vi "Facade.vi"(0 "Data In":T4, 2 "Display State In":T2, 3 "Container State":T3) -> (6 "Data Out":T4, 7 "Display State Out":T2, 8 "Action":T1)   [LabVIEW 2019, in "XTextCode.xctl"]
uses:
  XTextCode.xctl
  Data.ctl
  <vilib>/_xctls/Container State.ctl
  State.ctl
  <vilib>/_xctls/Action.ctl
  <vilib>/_xctls/XControlSupport.lvlib
  System.Windows.Forms
panel:
  in  "RichTextBox":refnum<k24>(container)
types:
  T1 = typedef "XControlSupport.lvlib/Action.ctl" = cluster{"Data Changed?":bool, "State Changed?":bool, "Action Name":string}
  T2 = typedef "XTextCode.xctl/State.ctl" = cluster{"String":string}
  T3 = typedef "XControlSupport.lvlib/Container State.ctl" = cluster{"Indicator?":bool, "Run Mode?":bool, " Refnum":refnum<vi>}
  T4 = typedef "XTextCode.xctl/Data.ctl" = string
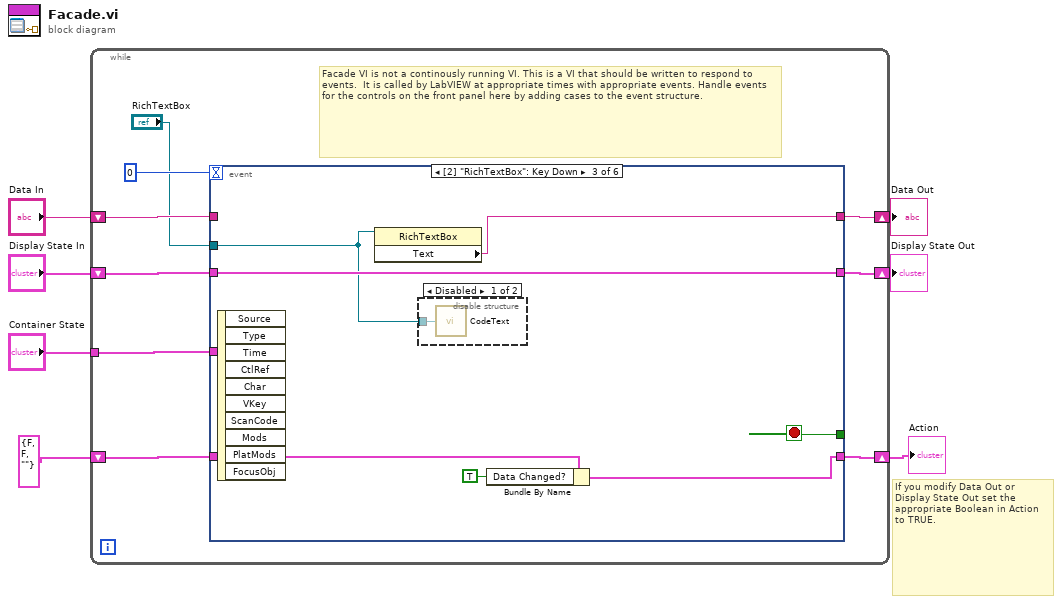
[diagram p0: block diagram]
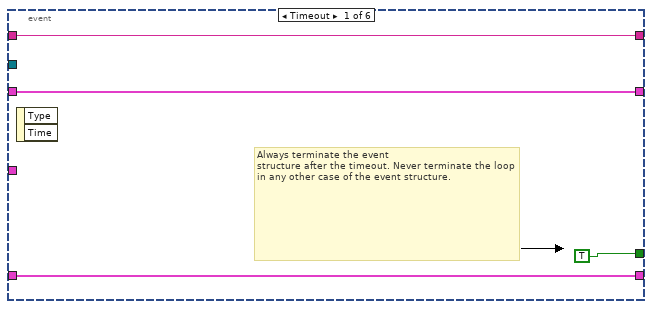
[diagram p2: hidden frame]
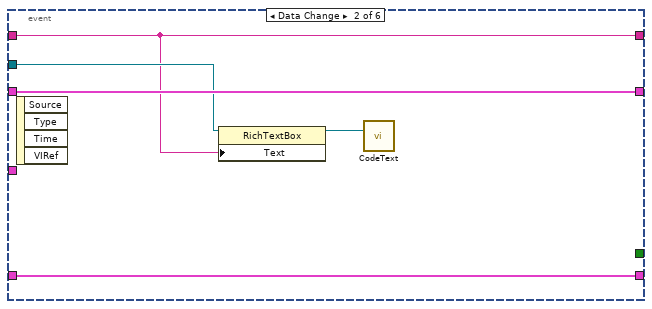
[diagram p3: hidden frame]
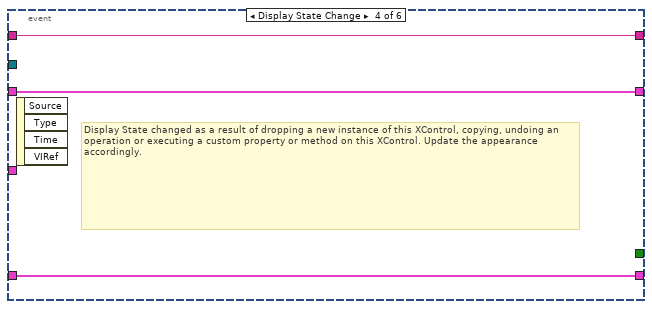
[diagram p5: hidden frame]
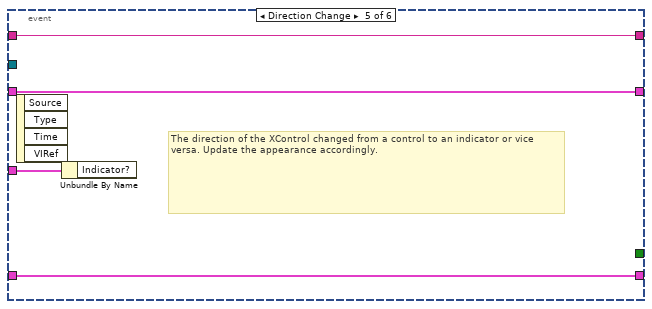
[diagram p6: hidden frame]
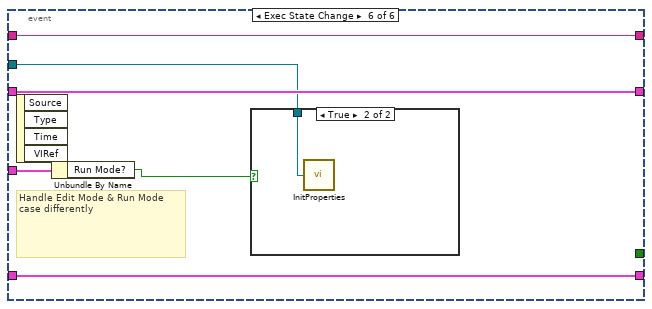
[diagram p7: hidden frame]
diagram:
  # "If you modify Data Out or\nDisplay State Out set the\nappropriate Boolean in Action\nto TRUE."
  n1 = while {
    shift-right: [w16] -> w4
    shift-left: "Display State In" -> [w17]
    tunnel: "Container State" -> [w13]
    shift-right: [w11] -> w7
    shift-left: "Data In" -> [w12]
    shift-right: [w9] -> w2
    shift-left: T1 {"Data Changed?"=FALSE, "State Changed?"=FALSE, "Action Name"=""} ("Action") -> [w10]
    stop <- w15 stop-if-true
    # "Facade VI is not a continously running VI. This is a VI that should be written to respond to events.  It is called by LabVIEW at appropriate times with appropriate events. Handle events for the controls on the front panel here by adding cases to the event structure."
    n2 = event shown="[2] \"RichTextBox\": Key Down" {
      selector: _ -> [_ _ _ _ _ _]
      dyn-events: _ -> [_ _ _ _ _ _]
      timeout: 0 -> [_ _ _ _ _ _]
      tunnel: w17 -> [w19 w26 w32 w36 w39 w45]
      tunnel: [w19 w26 w32 w36 w39 w45] -> w16
      tunnel: [TRUE _ _ _ _ _] -> w15
      tunnel: w13 -> [_ _ _ _ w40 w46]
      tunnel: w12 -> [w18 w23 _ w35 w38 w44]
      tunnel: [w18 w23 w30 w35 w38 w44] -> w11
      tunnel: [w20 w25 w28 w34 w37 w43] -> w9
      tunnel: w10 -> [w20 w25 w29 w34 w37 w43]
      tunnel: "RichTextBox" -> [_ w24 w31 _ _ w41]
      event Timeout {
        # "Always terminate the event\nstructure after the timeout. Never terminate the loop in any other case of the event structure."
        n3 = event-data() -> ()  [unwired: 1 in, 2 out]
      }
      event Data Change {
        n4 = event-data() -> ()  [unwired: 1 in, 4 out]
        n5 = property class="RichTextBox"(reference=w24, "Text"=w23) -> (reference out=w22:refnum<k24>)  [unwired: 1 in, 1 out]
        n6 = call "CodeText.vi"("Seq script"=w22) -> ()
      }
      event "RichTextBox": Key Down {
        n7 = event-data() -> ()  [unwired: 1 in, 10 out]
        n8 = property class="RichTextBox"(reference=w31) -> ("Text"=w30:string)  [unwired: 1 in, 2 out]
        n9 = disable-structure shown="Disabled" {
          disable-tunnel: w31 -> [w33 _]
          frame Disabled {
            n10 = call "CodeText.vi"("Seq script"=w33) -> ()
          }
          frame Enabled {
          }
        }
        n11 = Bundle By Name(cluster=w29, "Data Changed?"=TRUE) -> (w28:T1)
      }
      event Display State Change {
        # "Display State changed as a result of dropping a new instance of this XControl, copying, undoing an operation or executing a custom property or method on this XControl. Update the appearance accordingly."
        n12 = event-data() -> ()  [unwired: 1 in, 4 out]
      }
      event Direction Change {
        # "The direction of the XControl changed from a control to an indicator or vice versa. Update the appearance accordingly."
        n13 = event-data() -> ()  [unwired: 1 in, 4 out]
        n14 = Unbundle By Name(w40) -> ()  [unwired: 1 out]
      }
      event Exec State Change {
        # "Handle Edit Mode & Run Mode\ncase differently"
        n15 = event-data() -> ()  [unwired: 1 in, 4 out]
        n16 = Unbundle By Name(w46) -> ("Run Mode?"=w42:bool)
        n17 = case shown="True" w42 {
          tunnel: w41 -> [_ w47]
          frame False {
          }
          frame True {
            n18 = call "InitProperties.vi"("reference"=w47) -> ()
          }
        }
      }
    }
  }
  "Display State Out" <- w4
  "Data Out" <- w7
  "Action" <- w2
